vi "RP Scale.vi"(5 "Number of stages":i32=6, 6 "EEPROM offset":i32=78, 7 "Decimation":u32=1, 9 "EEPROM range":u32=45870551, 10 "Signal bits":i32=14, 11 "Range":dbl=1.0 format="%#_6eV") -> (1 "y intersept":dbl, 2 "Calibrated slope":dbl, 3 "Slope":dbl)   [LabVIEW 2016]
panel:
  out "Calibrated range":dbl
  out "x << y":i32
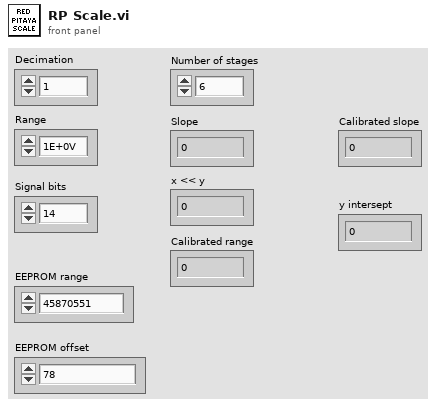
[diagram p1: front panel]
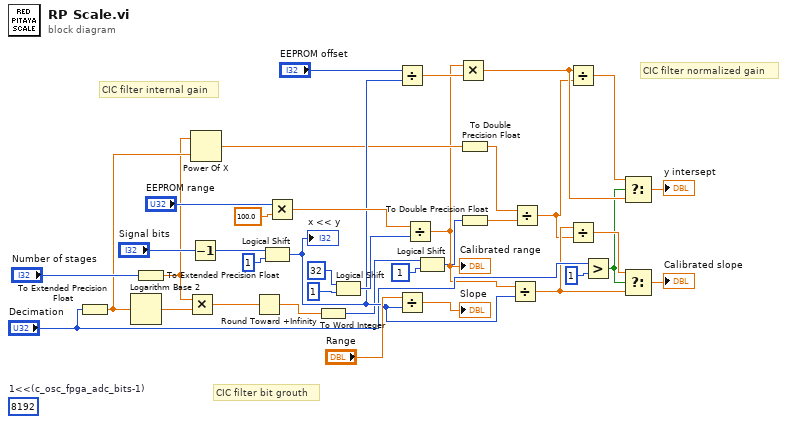
[diagram p0: block diagram]
diagram:
  (unwired) 8192  # 1<<(c_osc_fpga_adc_bits-1)
  # "CIC filter normalized gain"
  # "CIC filter internal gain"
  # "CIC filter bit grouth"
  n1 = To Extended Precision Float(1:"Decimation") -> (0:w19:ext)
  n2 = Logarithm Base 2(1:w19) -> (0:w17:ext)
  n3 = To Extended Precision Float(1:"Number of stages") -> (0:w18:ext)
  n4 = Multiply(x=w18, y=w17) -> (x*y=w14:ext)
  n5 = Decrement(x="Signal bits") -> (x-1=w37:i32)
  n6 = Power Of X(1:w19, 2:w18) -> (0:w11:ext)
  n7 = Round Toward +Infinity(x=w14) -> (ceil(x): smallest int >= x=w16:ext)
  n8 = Logical Shift(y=w37, x=1) -> (x << y=w23:i32)
  "x << y" <- w23
  n9 = Multiply(x="EEPROM range", y=100.0) -> (x*y=w28:dbl)
  n10 = To Word Integer(number=w16) -> (16bit integer=w13:i16)
  n11 = Logical Shift(y=i16 32, x=u64 1) -> (x << y=w27:u64)
  n12 = Divide(x="EEPROM offset", y=w23) -> (x/y=w25:dbl)
  n13 = Divide(x="Range", y=w23) -> (x/y=→"Slope":dbl)
  n14 = Divide(x=w28, y=w27) -> (x/y=w2:dbl)
  "Calibrated range" <- w2
  n15 = Logical Shift(y=w13, x=u64 1) -> (x << y=w12:u64)
  n16 = Multiply(x=w2, y=w25) -> (x*y=w24:dbl)
  n17 = To Double Precision Float(number=w11) -> (double precision float=w10:dbl)
  n18 = To Double Precision Float(number=w12) -> (double precision float=w9:dbl)
  n19 = Divide(x=w2, y=w23) -> (x/y=w5:dbl)
  n20 = Divide(x=w10, y=w9) -> (x/y=w4:dbl)
  n21 = Divide(x=w24, y=w4) -> (x/y=w8:dbl)
  n22 = Divide(x=w5, y=w4) -> (x/y=w7:dbl)
  n23 = Greater?(x="Decimation", y=u32 1) -> (0:w6:bool)
  n24 = Select(t=w8, s=w6, f=w24) -> (s? t:f=→"y intersept":dbl)
  n25 = Select(t=w7, s=w6, f=w5) -> (s? t:f=→"Calibrated slope":dbl)
